vi "simulation 0.1.vi"() -> ()   [LabVIEW 2019]
uses:
  <vilib>/Platform/TimedLoop/XDataNode/timing_clust.ctl
  <vilib>/Platform/TimedLoop/XDataNode/nitl_modes.ctl
  <vilib>/Platform/TimedLoop/XDataNode/wakeup.ctl
  <vilib>/Utility/inputDevices.llb/closeMouse.vi
  <vilib>/Utility/inputDevices.llb/closeKeyboard.vi
  <vilib>/Utility/inputDevices.llb/mouseAcquire.vi
  <vilib>/Utility/inputDevices.llb/keyboardAcquire.vi
  <vilib>/platform/TimedLoop/XDataNode/XDataNode.xnode
  <vilib>/Platform/TimedLoop/XDataNode/XDNodeRunTimeDep.lvlib
panel:
  in  "stop":bool
  in  "Tab Control":enum32{"map setting", " path planing"}(tab)
  in  "map range":T1
  in  "map setting path":path
  in  "map read":bool
  in  "map save":bool
  in  "wall settings":cluster{"Array":cluster{"X":dbl, "Y":dbl}[]}[](array[cluster])=[{"Array"=[{"X"=-258.0, "Y"=240.0}, {"X"=-258.0, "Y"=120.0}, {"X"=-261.0, "Y"=120.0}, {"X"=-261.0, "Y"=240.0}]}, {"Array"=[{"X"=-193.0, "Y"=60.5}, {"X"=-193.0, "Y"=177.0}, {"X"=-196.0, "Y"=177.0}, {"X"=-196.0, "Y"=60.5}]}, {"Array"=[{"X"=-341.0, "Y"=58.0}, {"X"=-59.5, "Y"=60.0}, {"X"=-59.5, "Y"=62.3}, {"X"=-341.0, "Y"=59.5}]}, {"Array"=[{"X"=-60.0, "Y"=59.5}, {"X"=-60.0, "Y"=180.0}, {"X"=-62.0, "Y"=180.0}, {"X"=-62.0, "Y"=59.5}]}, {"Array"=[{"X"=-61.5, "Y"=150.5}, {"X"=-61.6, "Y"=148.5}, {"X"=-101.5, "Y"=148.5}, {"X"=-101.5, "Y"=150.5}]}, {"Array"=[{"X"=-152.5, "Y"=150.5}, {"X"=-192.5, "Y"=150.5}, {"X"=-192.5, "Y"=148.5}, {"X"=-152.5, "Y"=148.5}]}]
  in  "Start zone":cluster{"X":dbl, "Y":dbl}
  in  "鍵盤靈敏度":u8(slide) scale=0.0..10.0
  in  "robot position":cluster{"X":dbl, "Y":dbl, "degree":dbl}
  in  "Auto?":bool
  in  "Device switch":enum16{"Mouse", "Keyboard"}(ring)
  in  "取點":bool
  in  "Path":T2(array[cluster])
  out "XY Graph":cluster{cluster{"X":dbl, "Y":dbl}[]}[](graph)
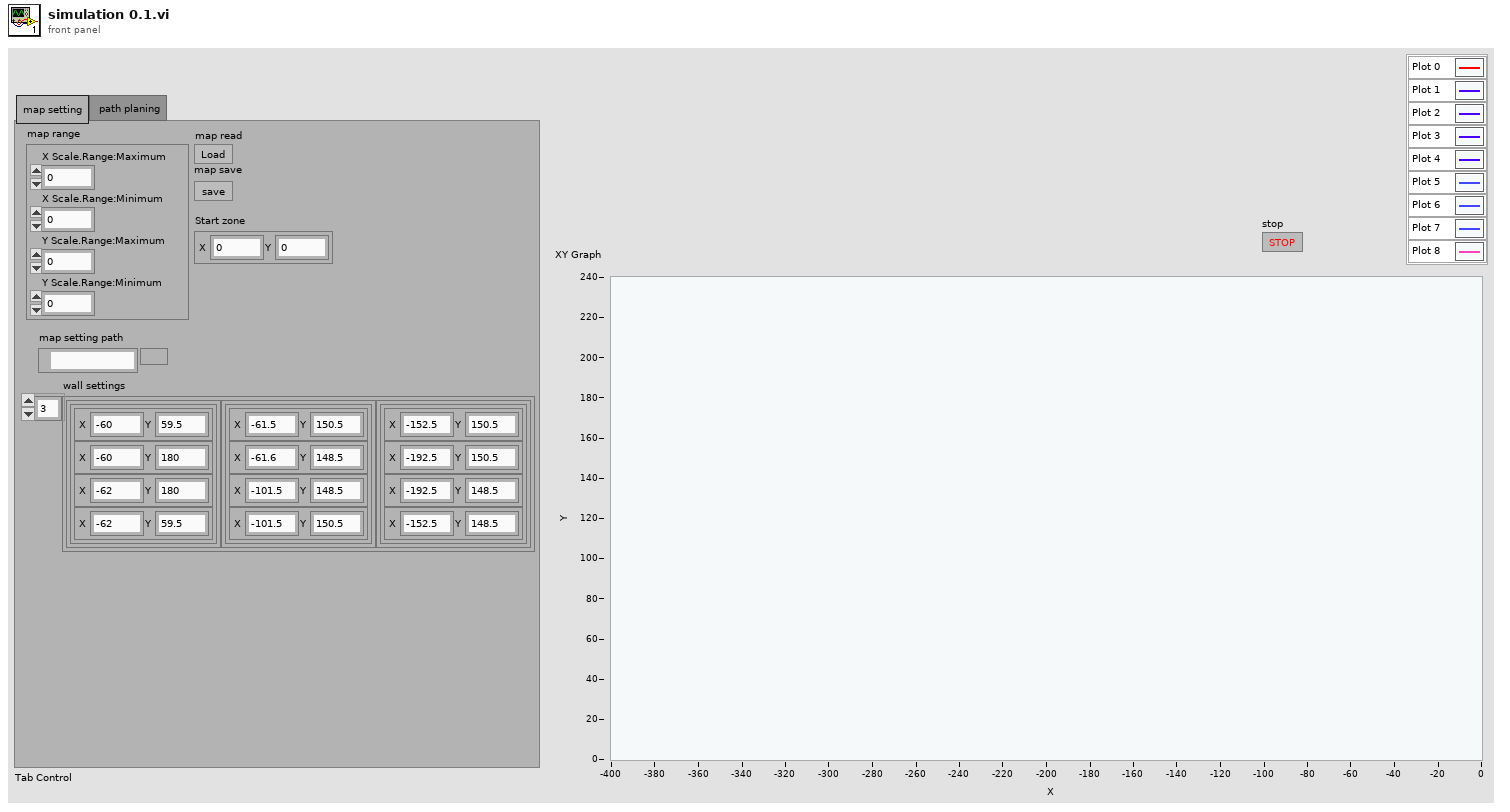
[diagram p1: front panel]
types:
  T1 = cluster{"X Scale.Range:Maximum":dbl, "X Scale.Range:Minimum":dbl, "Y Scale.Range:Maximum":dbl, "Y Scale.Range:Minimum":dbl}
  T2 = cluster{"X":dbl, "Y":dbl, "degree":dbl, "rotate":bool}[]
  T3 = typedef "XDNodeRunTimeDep.lvlib/timing_clust.ctl" = cluster{"Expected End [f-1]":u64, "Actual End [f-1]":u64, "Finished Late? [f-1]":bool, "Expected End [i-1]":u64, "Actual End [i-1]":u64, "Finished Late? [i-1]":bool, "Expected Start [i]":u64, "Actual Start [i]":u64, "Expected Start [f]":u64, "Actual Start [f]":u64, "Source Name":string, "Structure Name":string, "Period":i64, "Deadline":i64, "Offset":i64, "Start":i64, "Priority":i32, "Timeout":i32, "Mode":T4, "Wakeup Reason":T5, "Error":errorcluster, "Source Type":string, "Secondary Source Type":string, "Global End Time":u64, "Global Start Time":u64, "Frame Duration":u64, "Iteration Duration":u64, "Assigned CPU":i32, "I/O Scan Engine Mode":u32}
  T4 = typedef "XDNodeRunTimeDep.lvlib/nitl_modes.ctl" = enum32{"No Change", "Process missed periods, maintain original phase", "Discard missed periods, maintain original phase", "Process missed periods, ignore original phase", "Discard missed periods, ignore original phase"}
  T5 = typedef "XDNodeRunTimeDep.lvlib/wakeup.ctl" = enum32{"Normal", "Aborted", "Asynchronous wakeup", "Timing source error", "Timed loop error", "Timeout"}
  T6 = cluster{"axis info":cluster{"Horizontal":i32, "Vertical":i32, "Scrolling":i32}, "button info":cluster{"button 1":bool, "button 2":bool, "button 3":bool, "button 4":bool}}
  T7 = enum16{"close", "start keyboard", "start mouse", "output"}
  T8 = enum16{"0", "1", "2", "3", "4", "5", "6", "7", "8", "9", "A", "B", "C", "D", "E", "F", "G", "H", "I", "J", "K", "L", "M", "N", "O", "P", "Q", "R", "S", "T", "U", "V", "W", "X", "Y", "Z", "F1", "F2", "F3", "F4", "F5", "F6", "F7", "F8", "F9", "F10", "F11", "F12", "F13", "F14", "F15", "ADD", "BACK", "BACKSLASH", "CAPITAL", "COMMA", "DECIMAL", "DELETE", "DIVIDE", "DOWN", "END", "EQUALS", "ESCAPE", "GRAVE (`)", "HOME", "INSERT", "LBRACKET", "LCONTROL", "LEFT", "L ALT", "LSHIFT", "LWIN", "MINUS", "MULTIPLY", "NEXT", "NUMLOCK", "NUMPAD_0", "NUMPAD_1", "NUMPAD_2", "NUMPAD_3", "NUMPAD_4", "NUMPAD_5", "NUMPAD_6", "NUMPAD_7", "NUMPAD_8", "NUMPAD_9", "PAUSE", "PERIOD", "PRIOR (PG UP)", "RBRACKET", "RCONTROL", "RETURN", "RIGHT", "R ALT", "RSHIFT", "RWIN", "SCROLL", "SEMICOLON", "SLASH", "SPACE", "SUBTRACT", "TAB", "UP", "ENTER (num pad)", "' (quote)"}[]
  T9 = cluster{"Horizontal":i32, "Vertical":i32, "Scrolling":i32}
  T10 = cluster{"button 1":bool, "button 2":bool, "button 3":bool, "button 4":bool}
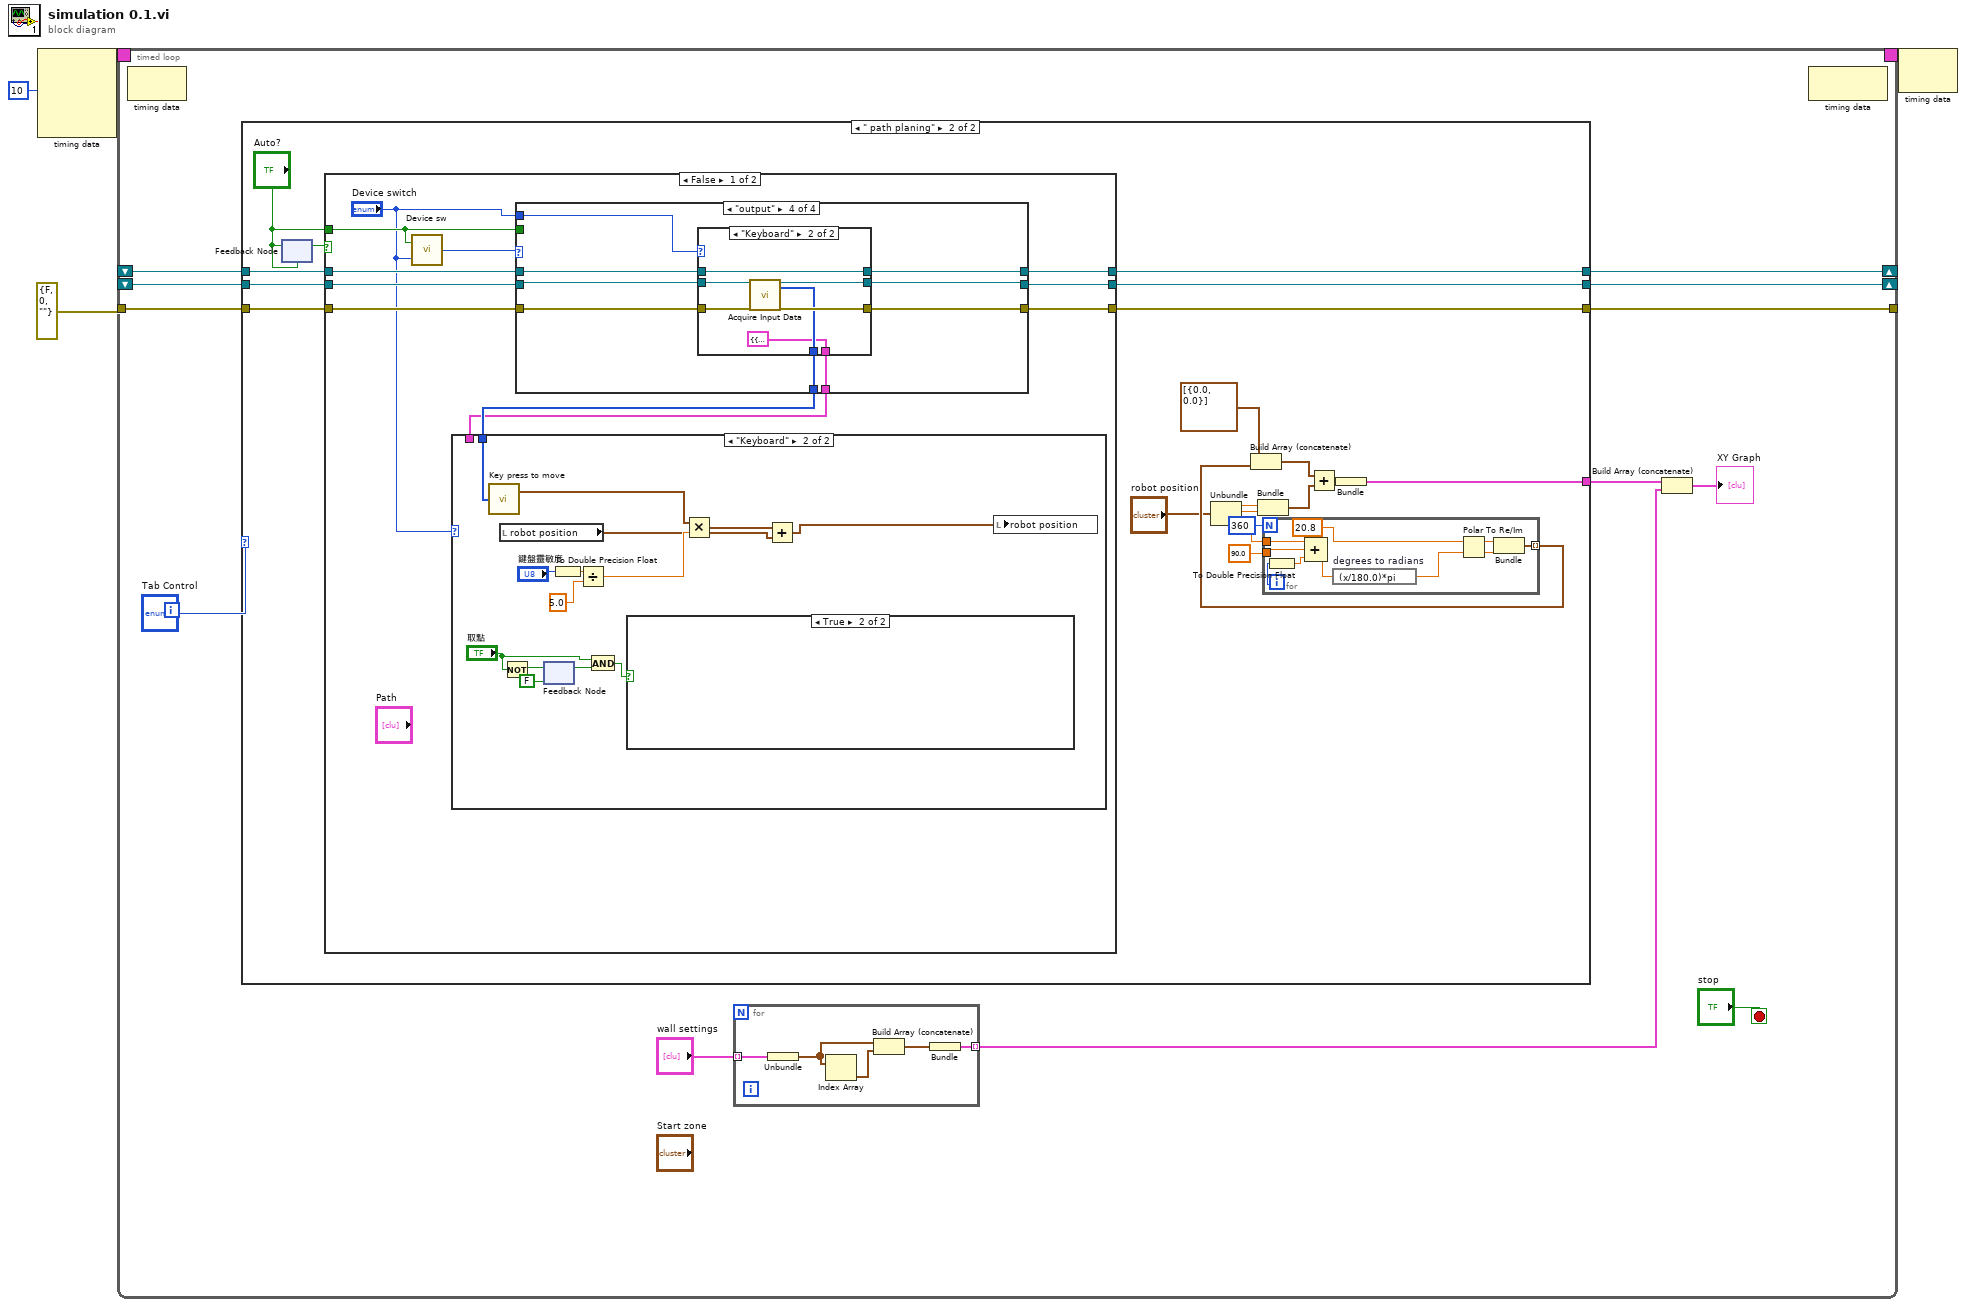
[diagram p0: block diagram]
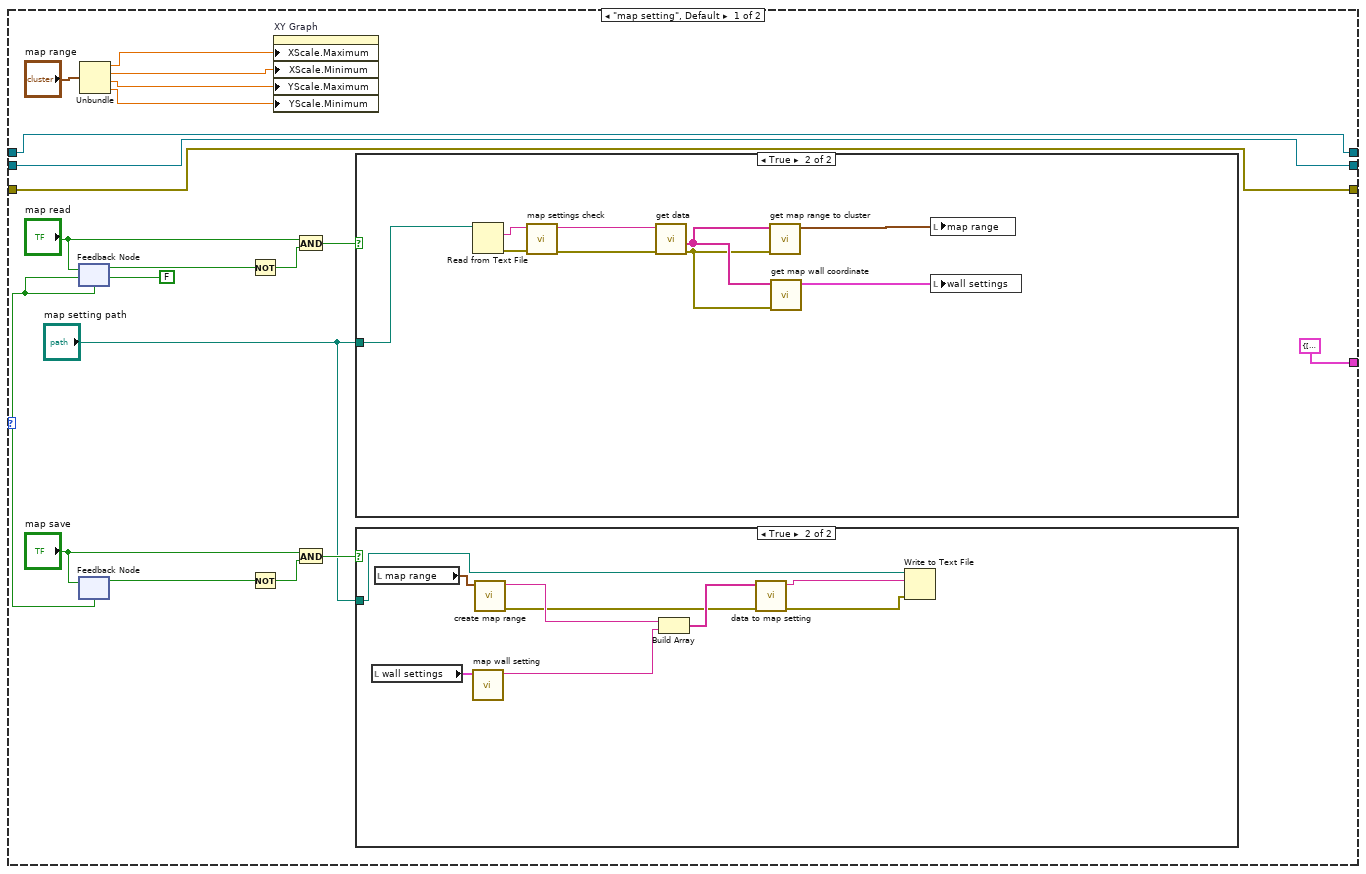
[diagram p2: hidden frame]
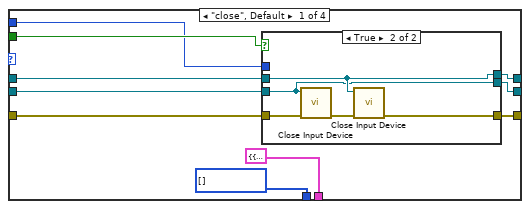
[diagram p7: hidden frame]
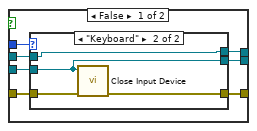
[diagram p8: hidden frame]
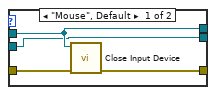
[diagram p9: hidden frame]
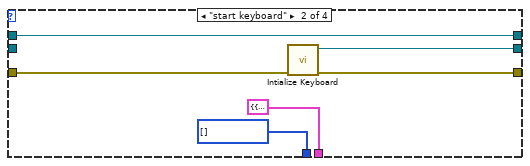
[diagram p10: hidden frame]
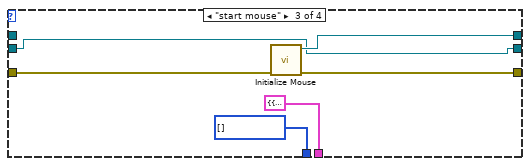
[diagram p11: hidden frame]
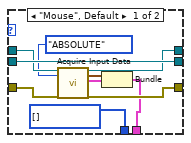
[diagram p12: hidden frame]
diagram:
  n1 = node-c288(i64 10 ("Period")) -> (w4:T3)  [unwired: 3 in]
  n2 = timed-loop {
    timing: w4 -> [_]
    timing-out: [_] -> w3
    shift-right: [w7] -> _
    shift-left: _ -> [w5]
    shift-right: [w8] -> _
    shift-left: _ -> [w6]
    tunnel: errorcluster {"status"=FALSE, "code"=0, "source"=""} ("error constant") -> [w9]
    tunnel: [w10] -> _
    stop <- "stop" stop-if-true
    n3 = node-c288() -> ()  [unwired: 1 in, 1 out]
    n4 = case shown="\" path planing\"" "Tab Control" {
      tunnel: [cluster{cluster{"X":dbl, "Y":dbl}[]} {[{"X"=0.0, "Y"=0.0}]} ("element") w74] -> w11
      tunnel: [w26 w68] -> w10
      tunnel: w9 -> [w26 w67]
      tunnel: [w25 w66] -> w8
      tunnel: [w24 w65] -> w7
      tunnel: w6 -> [w25 w64]
      tunnel: w5 -> [w24 w63]
      frame "map setting", Default {
        w28 = FALSE
        n5 = feedback #1(w28) -> (w30:bool)
        n6 = feedback-in #1("map read") -> ()
        n7 = feedback #2(w28) -> (w33:bool)
        n8 = feedback-in #2("map save") -> ()
        n9 = Unbundle("map range") -> ("X Scale.Range:Maximum"=w42:dbl, "X Scale.Range:Minimum"=w41:dbl, "Y Scale.Range:Maximum"=w40:dbl, "Y Scale.Range:Minimum"=w39:dbl)
        n10 = Not(x=w30) -> (.not. x?=w29:bool)
        n11 = Not(x=w33) -> (.not. x?=w34:bool)
        n12 = property on="XY Graph" class="XYGraph (strict)"("XScale.Maximum"=w42, "XScale.Minimum"=w41, "YScale.Maximum"=w40, "YScale.Minimum"=w39) -> ()  [unwired: 2 in, 2 out]
        n13 = And(x="map read", y=w29) -> (x .and. y?=w32:bool)
        n14 = And(x="map save", y=w34) -> (x .and. y?=w37:bool)
        n15 = case shown="True" w32 {
          tunnel: "map setting path" -> [_ w56]
          frame False {
          }
          frame True {
            n16 = Read from Text File(file (use dialog)=w56) -> (text=w59:string, error out=w60:errorcluster)  [unwired: 3 in, 2 out]
            n17 = call "map settings check.vi"("error in (no error)"=w60, "JSON in"=w59) -> ("error out"=w58:errorcluster, "JSON out"=w55:string)  [unwired: 8 in]
            n18 = call "get data.vi"("error in (no error)"=w58, "JSON in"=w55) -> ("error out"=w53:errorcluster, "data array"=w54:string[])  [unwired: 6 in, 2 out]
            n19 = call "get map range to cluster.vi"("error in (no error)"=w53, "data array"=w54) -> ("map range"=w57:cluster{dbl, dbl, dbl, dbl})  [unwired: 8 in, 1 out]
            n20 = call "get map wall coordinate.vi"("error in (no error)"=w53, "data array"=w54) -> ("Array"=w52:cluster{cluster{"X":dbl, "Y":dbl}[]}[])  [unwired: 8 in, 1 out]
            n21 = local write "map range"(w57) -> ()
            n22 = local write "wall settings"(w52) -> ()
          }
        }
        n23 = case shown="True" w37 {
          tunnel: "map setting path" -> [_ w43]
          frame False {
          }
          frame True {
            n24 = local read "wall settings"() -> (w47:cluster{"Array":cluster{"X":dbl, "Y":dbl}[]}[])
            n25 = local read "map range"() -> (w51:T1)
            n26 = call "map wall setting.vi"("wall settings"=w47) -> ("<JSON>"=w46:string)  [unwired: 9 in, 1 out]
            n27 = call "create map range.vi"("map range"=w51) -> ("error out"=w48:errorcluster, "<JSON> map range"=w50:string)  [unwired: 9 in]
            n28 = Build Array(w50, w46) -> (w49:string[])
            n29 = call "data to map setting.vi"("error in (no error)"=w48, "data in"=w49) -> ("error out"=w44:errorcluster, "<JSON>"=w45:string)  [unwired: 8 in]
            n30 = Write to Text File(file (use dialog)=w43, text=w45, error in=w44) -> ()  [unwired: 1 in, 3 out]
          }
        }
      }
      frame " path planing" {
        n31 = feedback #3("Auto?") -> (w62:bool)
        n32 = feedback-in #3("Auto?") -> ()
        n33 = case shown="False" w62 {
          tunnel: [w91 w174] -> w68
          tunnel: w67 -> [w90 w174]
          tunnel: [w89 w175] -> w66
          tunnel: [w88 w176] -> w65
          tunnel: w64 -> [w87 w175]
          tunnel: w63 -> [w86 w176]
          tunnel: "Auto?" -> [w85 _]
          frame False {
            n34 = call "Device sw.vi"("Device switch"="Device switch", "Auto?"=w85) -> ("output state"=w84:T7)
            n35 = case shown="\"output\"" w84 {
              tunnel: w90 -> [w113 w141 w147 w156]
              tunnel: [w110 w140 w146 w153] -> w91
              tunnel: [w107 w139 w142 w152] -> w89
              tunnel: [w106 w136 w145 w151] -> w88
              tunnel: w87 -> [w111 _ w142 w154]
              tunnel: w86 -> [w109 w136 _ w150]
              tunnel: "Device switch" -> [w108 _ _ w155]
              tunnel: [T6 {"axis info"={"Horizontal"=0, "Vertical"=0, "Scrolling"=0}, "button info"={"button 1"=FALSE, "button 2"=FALSE, "button 3"=FALSE, "button 4"=FALSE}} T6 {"axis info"={"Horizontal"=0, "Vertical"=0, "Scrolling"=0}, "button info"={"button 1"=FALSE, "button 2"=FALSE, "button 3"=FALSE, "button 4"=FALSE}} T6 {"axis info"={"Horizontal"=0, "Vertical"=0, "Scrolling"=0}, "button info"={"button 1"=FALSE, "button 2"=FALSE, "button 3"=FALSE, "button 4"=FALSE}} w149] -> w81
              tunnel: [w114 w137 w143 w148] -> w82
              tunnel: w85 -> [w112 _ _ _]
              frame "close", Default {
                w114 = T8 [] items=["0", "1", "2", "3", "4", "5", "6", "7", "8", "9", "A", "B", "C", "D", "E", "F", "G", "H", "I", "J", "K", "L", "M", "N", "O", "P", "Q", "R", "S", "T", "U", "V", "W", "X", "Y", "Z", "F1", "F2", "F3", "F4", "F5", "F6", "F7", "F8", "F9", "F10", "F11", "F12", "F13", "F14", "F15", "ADD", "BACK", "BACKSLASH", "CAPITAL", "COMMA", "DECIMAL", "DELETE", "DIVIDE", "DOWN", "END", "EQUALS", "ESCAPE", "GRAVE (`)", "HOME", "INSERT", "LBRACKET", "LCONTROL", "LEFT", "L ALT", "LSHIFT", "LWIN", "MINUS", "MULTIPLY", "NEXT", "NUMLOCK", "NUMPAD_0", "NUMPAD_1", "NUMPAD_2", "NUMPAD_3", "NUMPAD_4", "NUMPAD_5", "NUMPAD_6", "NUMPAD_7", "NUMPAD_8", "NUMPAD_9", "PAUSE", "PERIOD", "PRIOR (PG UP)", "RBRACKET", "RCONTROL", "RETURN", "RIGHT", "R ALT", "RSHIFT", "RWIN", "SCROLL", "SEMICOLON", "SLASH", "SPACE", "SUBTRACT", "TAB", "UP", "ENTER (num pad)", "' (quote)"] ("keys pressed")
                n36 = case shown="True" w112 {
                  tunnel: w113 -> [w121 w135]
                  tunnel: w111 -> [w120 w131]
                  tunnel: [w119 w133] -> w110
                  tunnel: w109 -> [w116 w132]
                  tunnel: w108 -> [w122 _]
                  tunnel: [w118 w131] -> w107
                  tunnel: [w117 w132] -> w106
                  frame False {
                    n37 = case shown="\"Keyboard\"" w122 {
                      tunnel: w121 -> [w126 w130]
                      tunnel: w120 -> [w123 w128]
                      tunnel: [w125 w129] -> w119
                      tunnel: [w123 w128] -> w118
                      tunnel: [w124 w127] -> w117
                      tunnel: w116 -> [w124 w127]
                      frame "Mouse", Default {
                        n38 = call-poly <vilib>:"Close Input Device.vi"("error in (no error)"=w126, "device ID"=w124) -> ("error out"=w125:errorcluster)  [unwired: 8 in]
                      }
                      frame "Keyboard" {
                        n39 = call-poly <vilib>:"Close Input Device.vi"("error in (no error)"=w130, "device ID"=w128) -> ("error out"=w129:errorcluster)  [unwired: 8 in]
                      }
                    }
                  }
                  frame True {
                    n40 = call-poly <vilib>:"Close Input Device.vi"("error in (no error)"=w135, "device ID"=w131) -> ("error out"=w134:errorcluster)  [unwired: 8 in]
                    n41 = call-poly <vilib>:"Close Input Device.vi"("error in (no error)"=w134, "device ID"=w132) -> ("error out"=w133:errorcluster)  [unwired: 8 in]
                  }
                }
              }
              frame "start keyboard" {
                w137 = T8 [] items=["0", "1", "2", "3", "4", "5", "6", "7", "8", "9", "A", "B", "C", "D", "E", "F", "G", "H", "I", "J", "K", "L", "M", "N", "O", "P", "Q", "R", "S", "T", "U", "V", "W", "X", "Y", "Z", "F1", "F2", "F3", "F4", "F5", "F6", "F7", "F8", "F9", "F10", "F11", "F12", "F13", "F14", "F15", "ADD", "BACK", "BACKSLASH", "CAPITAL", "COMMA", "DECIMAL", "DELETE", "DIVIDE", "DOWN", "END", "EQUALS", "ESCAPE", "GRAVE (`)", "HOME", "INSERT", "LBRACKET", "LCONTROL", "LEFT", "L ALT", "LSHIFT", "LWIN", "MINUS", "MULTIPLY", "NEXT", "NUMLOCK", "NUMPAD_0", "NUMPAD_1", "NUMPAD_2", "NUMPAD_3", "NUMPAD_4", "NUMPAD_5", "NUMPAD_6", "NUMPAD_7", "NUMPAD_8", "NUMPAD_9", "PAUSE", "PERIOD", "PRIOR (PG UP)", "RBRACKET", "RCONTROL", "RETURN", "RIGHT", "R ALT", "RSHIFT", "RWIN", "SCROLL", "SEMICOLON", "SLASH", "SPACE", "SUBTRACT", "TAB", "UP", "ENTER (num pad)", "' (quote)"] ("keys pressed")
                n42 = call <vilib>:"Intialize Keyboard.vi"("error in (no error)"=w141) -> ("error out"=w140:errorcluster, "device ID"=w139:refnum<k1>)  [unwired: 9 in]
              }
              frame "start mouse" {
                w143 = T8 [] items=["0", "1", "2", "3", "4", "5", "6", "7", "8", "9", "A", "B", "C", "D", "E", "F", "G", "H", "I", "J", "K", "L", "M", "N", "O", "P", "Q", "R", "S", "T", "U", "V", "W", "X", "Y", "Z", "F1", "F2", "F3", "F4", "F5", "F6", "F7", "F8", "F9", "F10", "F11", "F12", "F13", "F14", "F15", "ADD", "BACK", "BACKSLASH", "CAPITAL", "COMMA", "DECIMAL", "DELETE", "DIVIDE", "DOWN", "END", "EQUALS", "ESCAPE", "GRAVE (`)", "HOME", "INSERT", "LBRACKET", "LCONTROL", "LEFT", "L ALT", "LSHIFT", "LWIN", "MINUS", "MULTIPLY", "NEXT", "NUMLOCK", "NUMPAD_0", "NUMPAD_1", "NUMPAD_2", "NUMPAD_3", "NUMPAD_4", "NUMPAD_5", "NUMPAD_6", "NUMPAD_7", "NUMPAD_8", "NUMPAD_9", "PAUSE", "PERIOD", "PRIOR (PG UP)", "RBRACKET", "RCONTROL", "RETURN", "RIGHT", "R ALT", "RSHIFT", "RWIN", "SCROLL", "SEMICOLON", "SLASH", "SPACE", "SUBTRACT", "TAB", "UP", "ENTER (num pad)", "' (quote)"] ("keys pressed")
                n43 = call <vilib>:"Initialize Mouse.vi"("error in (no error)"=w147) -> ("error out"=w146:errorcluster, "device ID"=w145:refnum<k1>)  [unwired: 9 in]
              }
              frame "output" {
                n44 = case shown="\"Keyboard\"" w155 {
                  tunnel: w156 -> [w165 w173]
                  tunnel: w154 -> [w166 w172]
                  tunnel: [w164 w171] -> w153
                  tunnel: [w166 w170] -> w152
                  tunnel: [w163 w167] -> w151
                  tunnel: w150 -> [w162 w167]
                  tunnel: [w158 T6 {"axis info"={"Horizontal"=0, "Vertical"=0, "Scrolling"=0}, "button info"={"button 1"=FALSE, "button 2"=FALSE, "button 3"=FALSE, "button 4"=FALSE}}] -> w149
                  tunnel: [w157 w169] -> w148
                  frame "Mouse", Default {
                    w157 = T8 [] items=["0", "1", "2", "3", "4", "5", "6", "7", "8", "9", "A", "B", "C", "D", "E", "F", "G", "H", "I", "J", "K", "L", "M", "N", "O", "P", "Q", "R", "S", "T", "U", "V", "W", "X", "Y", "Z", "F1", "F2", "F3", "F4", "F5", "F6", "F7", "F8", "F9", "F10", "F11", "F12", "F13", "F14", "F15", "ADD", "BACK", "BACKSLASH", "CAPITAL", "COMMA", "DECIMAL", "DELETE", "DIVIDE", "DOWN", "END", "EQUALS", "ESCAPE", "GRAVE (`)", "HOME", "INSERT", "LBRACKET", "LCONTROL", "LEFT", "L ALT", "LSHIFT", "LWIN", "MINUS", "MULTIPLY", "NEXT", "NUMLOCK", "NUMPAD_0", "NUMPAD_1", "NUMPAD_2", "NUMPAD_3", "NUMPAD_4", "NUMPAD_5", "NUMPAD_6", "NUMPAD_7", "NUMPAD_8", "NUMPAD_9", "PAUSE", "PERIOD", "PRIOR (PG UP)", "RBRACKET", "RCONTROL", "RETURN", "RIGHT", "R ALT", "RSHIFT", "RWIN", "SCROLL", "SEMICOLON", "SLASH", "SPACE", "SUBTRACT", "TAB", "UP", "ENTER (num pad)", "' (quote)"] ("keys pressed")
                    n45 = call-poly <vilib>:"Acquire Input Data.vi"("device ID"=w162, "key mode"=enum16{"RELATIVE", "ABSOLUTE"}."ABSOLUTE", "error in (no error)"=w165) -> ("device ID"=w163:refnum<k1>, "axis info"=w160:T9, "button info"=w159:T10, "error out"=w164:errorcluster)  [unwired: 13 in]
                    n46 = Bundle("axis info"=w160, "button info"=w159) -> (w158:T6)  [unwired: 1 in]
                  }
                  frame "Keyboard" {
                    n47 = call-poly <vilib>:"Acquire Input Data.vi"("device ID"=w172, "error in (no error)"=w173) -> ("device ID"=w170:refnum<k1>, "keys pressed"=w169:T8, "error out"=w171:errorcluster)  [unwired: 15 in]
                  }
                }
              }
            }
            n48 = case shown="\"Keyboard\"" "Device switch" {
              tunnel: w82 -> [_ w105]
              tunnel: w81 -> [_ _]
              frame "Mouse", Default {
              }
              frame "Keyboard" {
                n49 = call "Key press to move.vi"("keys pressed"=w105) -> ("move"=w100:cluster{"X":dbl, "Y":dbl, "degree":dbl})  [unwired: 1 in]
                n50 = local read "robot position"() -> (w98:cluster{"X":dbl, "Y":dbl, "degree":dbl})
                n51 = Not(x="取點") -> (.not. x?=w96:bool)
                n52 = feedback #4(FALSE) -> (w94:bool)
                n53 = feedback-in #4(w96) -> ()
                n54 = To Double Precision Float(number="鍵盤靈敏度") -> (double precision float=w102:dbl)
                n55 = Divide(x=w102, y=5.0) -> (x/y=w101:dbl)
                n56 = And(x="取點", y=w94) -> (x .and. y?=w92:bool)
                n57 = case shown="True" w92 {
                  frame False {
                  }
                  frame True {
                  }
                }
                n58 = Multiply(x=w100, y=w101) -> (x*y=w99:cluster{"X":dbl, "Y":dbl, "degree":dbl})
                n59 = Add(x=w99, y=w98) -> (x+y=w97:cluster{"X":dbl, "Y":dbl, "degree":dbl})
                n60 = local write "robot position"(w97) -> ()
              }
            }
          }
          frame True {
          }
        }
        n61 = Unbundle("robot position") -> ("X"=w75:dbl, "Y"=w76:dbl, "degree"=w80:dbl)
        n62 = Bundle("X"=w75, "Y"=w76) -> (w70:cluster{"X":dbl, "Y":dbl})  [unwired: 1 in]
        n63 = for {
          N: 360 -> [_]
          tunnel: w80 -> [w186]
          tunnel: 90.0 -> [w183]
          tunnel: [w179] -> w78 mode=indexing
          i -> [w184]
          n64 = To Double Precision Float(number=w184) -> (double precision float=w185:dbl)
          n65 = Compound Arithmetic op=ADD(w186, w183, w185) -> (w180:dbl)
          n66 = expression code="(x/180.0)*pi" "degrees to radians"(w180) -> (w178:dbl)
          n67 = Polar To Re/Im(2:w178, 3:20.8 ("r")) -> (0:w177:dbl, 1:w181:dbl)
          n68 = Bundle(w181, w177) -> (w179:cluster{dbl, dbl})  [unwired: 1 in]
        }
        n69 = Build Array (concatenate)(cluster{dbl, dbl}[] [{0.0, 0.0}] ("element"), w78) -> (w71:cluster{dbl, dbl}[])
        n70 = Add(x=w71, y=w70) -> (x+y=w72:cluster{dbl, dbl}[])
        n71 = Bundle(w72) -> (w74:cluster{cluster{dbl, dbl}[]})  [unwired: 1 in]
      }
    }
    n72 = for {
      tunnel: "wall settings" -> [w20] mode=indexing
      tunnel: [w19] -> w12 mode=indexing
      n73 = Unbundle(w20) -> ("Array"=w22:cluster{"X":dbl, "Y":dbl}[])
      n74 = Index Array(array=w22) -> (element=w23:cluster{"X":dbl, "Y":dbl})  [unwired: 1 in]
      n75 = Build Array (concatenate)(w22, w23) -> (w21:cluster{"X":dbl, "Y":dbl}[])
      n76 = Bundle(w21) -> (w19:cluster{cluster{"X":dbl, "Y":dbl}[]})  [unwired: 1 in]
    }
    n77 = Build Array (concatenate)(w11, w12) -> (→"XY Graph":cluster{cluster{"X":dbl, "Y":dbl}[]}[])
    n78 = node-c288() -> ()  [unwired: 1 in, 1 out]
  }
  n79 = node-c288(w3) -> ()  [unwired: 1 out]
